vi "GoToPosAbs.vi"(8 "error in (no error)":errorcluster caption="entrée d'erreur (pas d'erreur)", 11 "UI SA en entrée":refnum<class "UI SmarAct.lvclass">) -> (0 "error out":errorcluster caption="sortie d'erreur", 3 "UI SA en sortie":refnum<class "UI SmarAct.lvclass">)   [LabVIEW 2024, in "UI SmarAct.lvclass"]
uses:
  UI SmarAct.lvclass
  UI SmarAct.lvclass/UI SmarAct.ctl
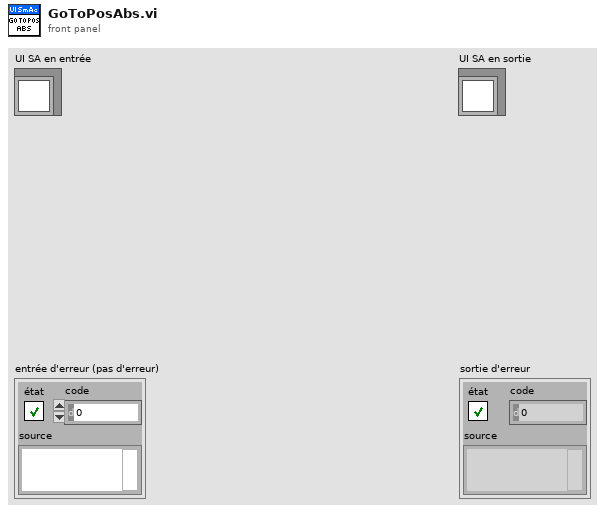
[diagram p1: front panel]
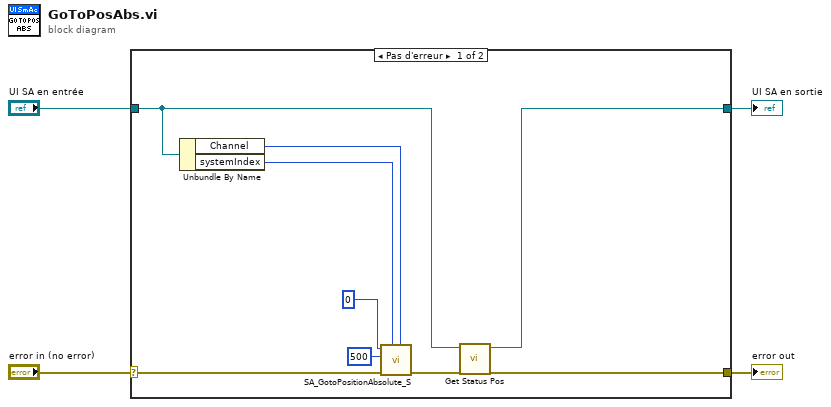
[diagram p0: block diagram]
diagram:
  n1 = case shown="Pas d'erreur" "error in (no error)" {
    selector: "error in (no error)" -> [w13 w15]
    tunnel: [w7 w15] -> w3
    tunnel: [w5 w14] -> w1
    tunnel: "UI SA en entrée" -> [w6 w14]
    frame No Error {
      n2 = Unbundle By Name(w6) -> ("Channel"=w12:u32, "systemIndex"=w11:u32)
      n3 = call <vilib>:"SA_GotoPositionAbsolute_S.vi"("channelIndex"=w12, "systemIndex"=w11, "error in (no error)"=w13, "holdTime"=u32 500, "position"=0) -> ("error out"=w8:errorcluster)  [unwired: 6 in]
      n4 = call "Get Status Pos.vi"("error in (no error)"=w8, "UI SA en entrée"=w6) -> ("error out"=w7:errorcluster, "UI SA en sortie"=w5:refnum<class "UI SmarAct.lvclass">)  [unwired: 8 in]
    }
    frame Error {
    }
  }
  "error out" <- w3
  "UI SA en sortie" <- w1
